vi "Complex Eigenvalues and Vectors.vi"(3 "output option":T1=1 items=["Eigenvalues", "Eigenvalues & Vectors"], 4 "matrix type":i32(ring) items=["General", "Hermitian"], 5 "Input Matrix":T2) -> (0 "error":i32, 1 "Eigenvectors":T2, 2 "Eigenvalues":cdb[](array[numeric]) format="%.2f")   [LabVIEW 2010, in "NI_AALPro.lvlib"]
doc: "Finds the eigenvalues and right eigenvectors of the square <B>Input Matrix</B>. Wire data to the <B>Input Matrix</B> input to determine the polymorphic instance to use or manually select the instance."
uses:
  NI_AALPro.lvlib
  ComplexMatrix.ctl
  Eigenvalue and Vectors Output Option.ctl
  lvanlys.dll
  NI_Matrix.lvlib
panel:
  # "Complex Eigenvalues and Vectors"
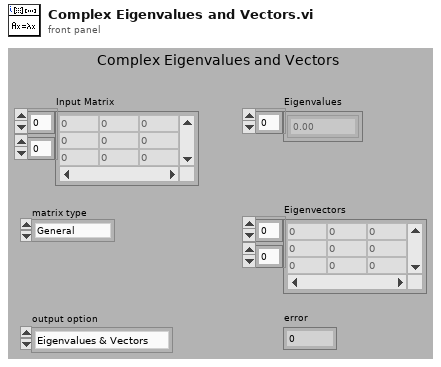
[diagram p1: front panel]
types:
  T1 = typedef "NI_AALPro.lvlib/Eigenvalue and Vectors Output Option.ctl" = i32
  T2 = typedef "NI_Matrix.lvlib/ComplexMatrix.ctl" = cdb[][]
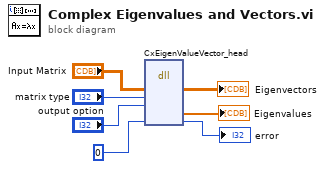
[diagram p0: block diagram]
diagram:
  n1 = dll-call lib="C:/Program Files/National Instruments/LabVIEW 2010/resource/lvanlys.*" fn="CxEigenValueVector_head"("aH"="Input Matrix", "mtype"="matrix type", "otype"="output option", "dsperr"=0) -> ("aH"=→"Eigenvectors":T2, "Eigenvalues"=→"Eigenvalues":cdb[], "dsperr"=→"error":i32)  [unwired: 7 in, 2 out]
